vi "Update Device.vi"(7 "Device":T9, 9 "Device State":T1={"Type"=enum."Mass Flow Controller", "Label"="", "User Tag"="", "MB_TCP session"=refnum, "Control State"={"Control Mode"=0, "Function"=enum."Downstream pressure", "FSetpoint"=0.0, "Flow Capacity Unit"="", "Setpoint Slope"=0, "P1Setpoint"=0.0, "P2Setpoint"=0.0}, "Measurement State"={"Fmeasure"=0.0, "P1measure"=0.0, "P2measure"=0.0}} {"Control State"."Control Mode" items=["Bus/RS232"=0, "FLOW-BUS slave"=2, "Valve close"=3, "Controller idle"=4, "Setpoint 100%"=7, "Valve fully open"=8, "Calibration mode"=9, "Setpoint 0%"=12, "RS232"=18, "Valve steering"=20, "Valve safe state"=22]}, 10 "MB_TCP session":refnum<class "MB_Master_TCP.lvclass">, 11 "Data Cluster":T7 {"Flexi-Flow Devices"."Control State"."Control Mode" items=["Bus/RS232"=0, "FLOW-BUS slave"=2, "Valve close"=3, "Controller idle"=4, "Setpoint 100%"=7, "Valve fully open"=8, "Calibration mode"=9, "Setpoint 0%"=12, "RS232"=18, "Valve steering"=20, "Valve safe state"=22]}) -> (3 "Data Cluster Out":T7 {"Flexi-Flow Devices"."Control State"."Control Mode" items=["Bus/RS232"=0, "FLOW-BUS slave"=2, "Valve close"=3, "Controller idle"=4, "Setpoint 100%"=7, "Valve fully open"=8, "Calibration mode"=9, "Setpoint 0%"=12, "RS232"=18, "Valve steering"=20, "Valve safe state"=22]})   [LabVIEW 2024, in "FlexiFlowInterface.lvlib"]
uses:
  FlexiFlowInterface.lvlib
  FlexiFlowDevice--enum.ctl
  Module Data--cluster.ctl
  Modbus TCP Connection Settings--cluster.ctl
  Modbus Flexi-Flow State--cluster.ctl
  <vilib>/Plasmionique/MB Master/MB_Master_TCP/MB_Master_TCP.lvclass
  Device Type--enum.ctl
  Modbus Flexi-Flow Controls--cluster.ctl
  Modbus Flexi-Flow API/Control Mode--enum.ctl
  Modbus Flexi-Flow API/Control Function Values--enum.ctl
  Modbus Flexi-Flow Measure State--cluster.ctl
  Modbus Flexi-Flow API/Bronkhorst Flexi-Flow ModbusTCP API.lvlib
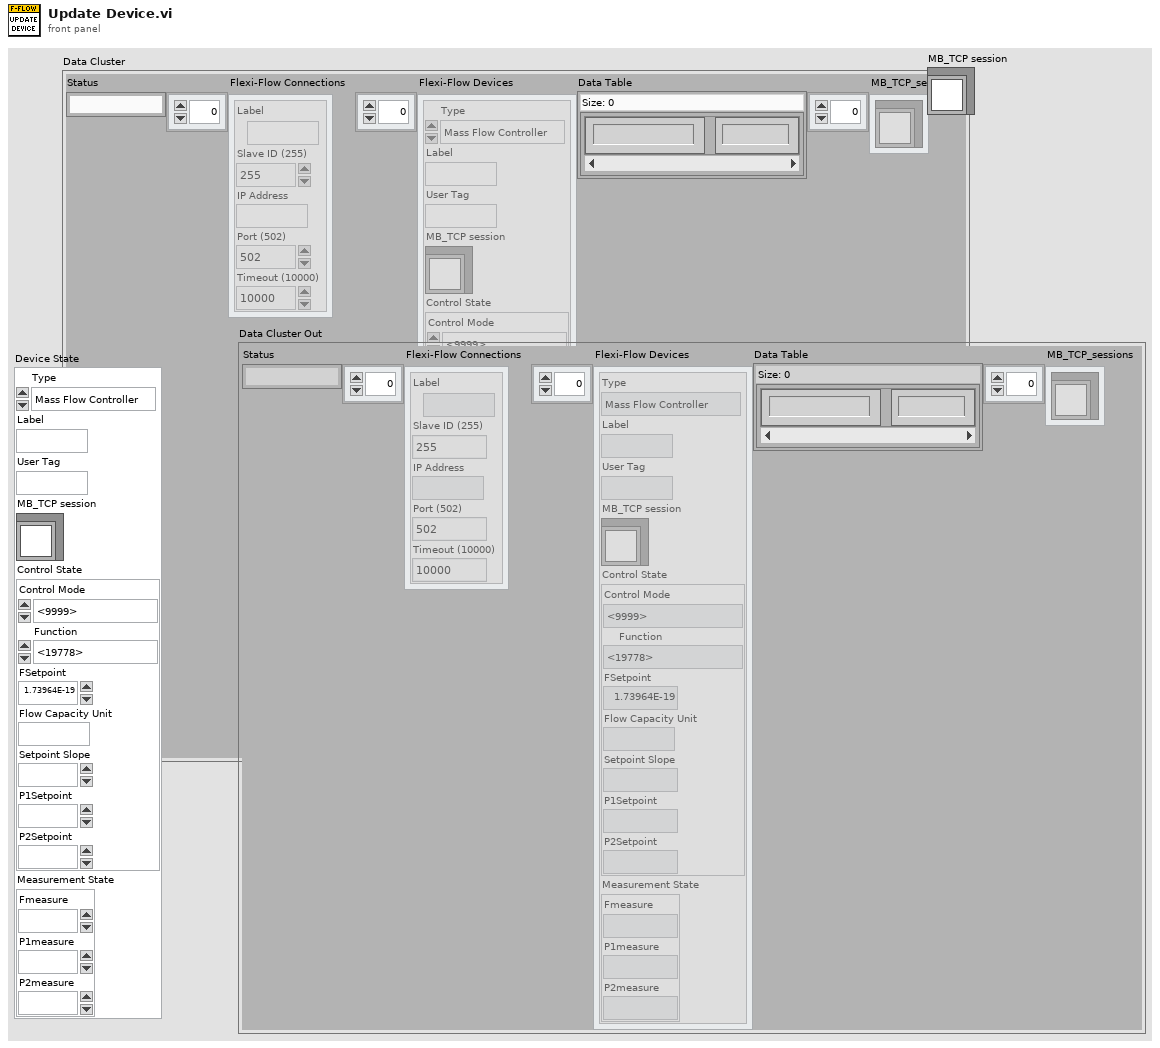
[diagram p1: front panel]
types:
  T1 = typedef "FlexiFlowInterface.lvlib/Modbus Flexi-Flow State--cluster.ctl" = cluster{"Type":T2, "Label":string, "User Tag":string, "MB_TCP session":refnum<class "MB_Master_TCP.lvclass">, "Control State":T3, "Measurement State":T6}
  T2 = typedef "FlexiFlowInterface.lvlib/Device Type--enum.ctl" = enum16{"Mass Flow Controller", "Mass Flow Meter"}
  T3 = typedef "FlexiFlowInterface.lvlib/Modbus Flexi-Flow Controls--cluster.ctl" = cluster{"Control Mode":T4, "Function":T5, "FSetpoint":sgl, "Flow Capacity Unit":string, "Setpoint Slope":u16, "P1Setpoint":sgl, "P2Setpoint":sgl}
  T4 = typedef "Bronkhorst Flexi-Flow ModbusTCP API.lvlib/Control Mode--enum.ctl" = u16
  T5 = typedef "Bronkhorst Flexi-Flow ModbusTCP API.lvlib/Control Function Values--enum.ctl" = enum16{"Flow", "Upstream pressure", "Downstream pressure", "Flow with upstream pressure limit", "Flow with downstream pressure limit", "Upstream pressure with flow limit", "Downstream pressure with flow limit"}
  T6 = typedef "FlexiFlowInterface.lvlib/Modbus Flexi-Flow Measure State--cluster.ctl" = cluster{"Fmeasure":dbl, "P1measure":sgl, "P2measure":sgl}
  T7 = typedef "FlexiFlowInterface.lvlib/Module Data--cluster.ctl" = cluster{"Status":string, "Flexi-Flow Connections":T8[], "Flexi-Flow Devices":T1[], "Data Table":map{string, dbl}, "MB_TCP_sessions":refnum<class "MB_Master_TCP.lvclass">[]}
  T8 = typedef "FlexiFlowInterface.lvlib/Modbus TCP Connection Settings--cluster.ctl" = cluster{"Label":string, "Slave ID (255)":u8, "IP Address":string, "Port (502)":u16, "Timeout (10000)":i32}
  T9 = typedef "FlexiFlowInterface.lvlib/FlexiFlowDevice--enum.ctl" = enum16{"Hydrogen Inlet", "Nitrogen Inlet", "Cathode Outlet", "Anode Outlet"}
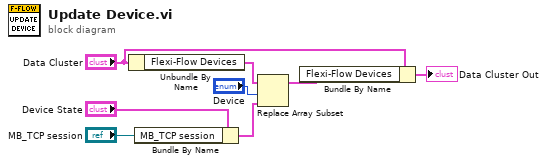
[diagram p0: block diagram]
diagram:
  n1 = Unbundle By Name("Data Cluster") -> ("Flexi-Flow Devices"=w8:T1[])
  n2 = Bundle By Name(cluster="Device State", "MB_TCP session"="MB_TCP session") -> (w2:T1)
  n3 = Replace Array Subset(array=w8, new element=w2, index="Device") -> (w5:T1[])
  n4 = Bundle By Name(cluster="Data Cluster", "Flexi-Flow Devices"=w5) -> (→"Data Cluster Out":T7)
